vi "Icon Header.vi"(9 "Add Border? (F)":bool, 10 "BG (0=Random)":u32(colorbox), 11 "Text":string) -> (2 "BG out":u32(colorbox), 3 "Color256":T1)   [LabVIEW 2018, in "Pkg.lvlib"]
uses:
  Pkg.lvlib
  <vilib>/picture/picture.llb/imagedata.ctl
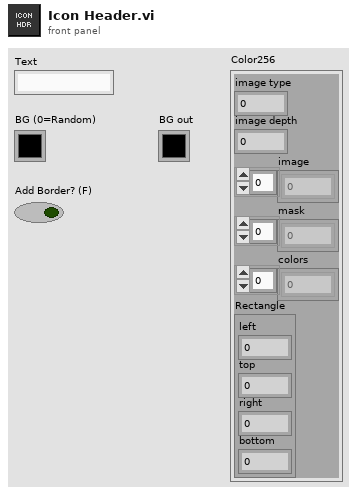
[diagram p1: front panel]
types:
  T1 = typedef "imagedata.ctl" = cluster{"image type":i32, "image depth":i32, "image":u8[], "mask":u8[], "colors":u32[], "Rectangle":cluster{"left":i16, "top":i16, "right":i16, "bottom":i16}}
  T2 = cluster{"left":i16, "top":i16, "right":i16, "bottom":i16}
  T3 = cluster{"Font Name:":string, "Size":i16, "Strikeout?":bool, "Italic?":bool, "Underline?":bool, "Outline?":bool, "Shadow?":bool, "Bold?":bool}
  T4 = enum16{"User-specified Font", "Application Font", "System Font", "Dialog Font"}
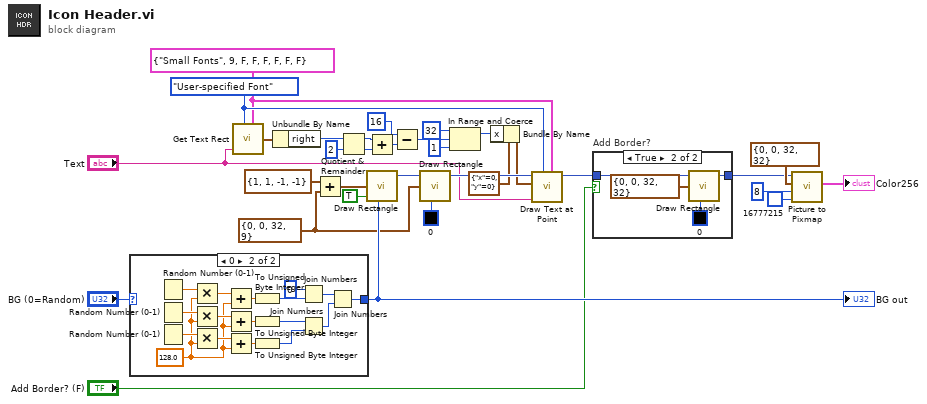
[diagram p0: block diagram]
diagram:
  w23 = T2 {"left"=0, "top"=0, "right"=32, "bottom"=9} ("rect")
  w20 = T3 {"Font Name:"="Small Fonts", "Size"=9, "Strikeout?"=FALSE, "Italic?"=FALSE, "Underline?"=FALSE, "Outline?"=FALSE, "Shadow?"=FALSE, "Bold?"=FALSE} ("[user-specified font]")
  w21 = T4."User-specified Font" ("desired font(Application)")
  n1 = case shown="0" "BG (0=Random)" {
    selector: "BG (0=Random)" -> [w33 _]
    tunnel: [w33 w38] -> w28
    frame Default {
    }
    frame 0 {
      w34 = 128.0 ("y")
      n2 = Random Number (0-1)() -> (number: 0 to 1=w49:dbl)
      n3 = Random Number (0-1)() -> (number: 0 to 1=w48:dbl)
      n4 = Random Number (0-1)() -> (number: 0 to 1=w45:dbl)
      n5 = Multiply(x=w49, y=w34) -> (x*y=w50:dbl)
      n6 = Multiply(x=w48, y=w34) -> (x*y=w47:dbl)
      n7 = Multiply(x=w45, y=w34) -> (x*y=w46:dbl)
      n8 = Add(x=w50, y=w34) -> (x+y=w35:dbl)
      n9 = Add(x=w47, y=w34) -> (x+y=w36:dbl)
      n10 = Add(x=w46, y=w34) -> (x+y=w37:dbl)
      n11 = To Unsigned Byte Integer(number=w35) -> (unsigned 8bit integer=w44:u8)
      n12 = To Unsigned Byte Integer(number=w36) -> (unsigned 8bit integer=w42:u8)
      n13 = To Unsigned Byte Integer(number=w37) -> (unsigned 8bit integer=w41:u8)
      n14 = Join Numbers(hi=u8 0, lo=w44) -> ((hi.lo)=w39:u16)
      n15 = Join Numbers(hi=w42, lo=w41) -> ((hi.lo)=w40:u16)
      n16 = Join Numbers(hi=w39, lo=w40) -> ((hi.lo)=w38:u32)
    }
  }
  "BG out" <- w28
  n17 = call <vilib>:"Get Text Rect.vi"("desired font(Application)"=w21, "text"="Text", "[user-specified font]"=w20) -> ("rect"=w19:T2)  [unwired: 6 in]
  n18 = Unbundle By Name(w19) -> ("right"=w9:i16)
  n19 = Add(x=T2 {"left"=1, "top"=1, "right"=-1, "bottom"=-1} ("rect"), y=w23) -> (x+y=w24:T2)
  n20 = Quotient & Remainder(x=w9, y=i16 2) -> (x-y*floor(x/y)=w6:i16, floor(x/y)=w12:i16)
  n21 = Add(x=w6, y=w12) -> (x+y=w7:i16)
  n22 = call <vilib>:"Draw Rectangle.vi"("rect"=w24, "fill?(F)"=TRUE, "color(black)"=w28) -> ("new picture"=w30:picture)  [unwired: 6 in]
  n23 = Subtract(x=i16 16 ("y"), y=w7) -> (x-y=w5:i16)
  n24 = call <vilib>:"Draw Rectangle.vi"("picture"=w30, "rect"=w23, "color(black)"=u32 0) -> ("new picture"=w22:picture)  [unwired: 6 in]
  n25 = In Range and Coerce(upper limit=i16 32, x=w5, lower limit=i16 1) -> (coerced(x)=w11:i16)  [unwired: 1 out]
  n26 = Bundle By Name(cluster=cluster{"x":i16, "y":i16} {"x"=0, "y"=0} ("origin"), "x"=w11) -> (w16:cluster{"x":i16, "y":i16})
  n27 = call <vilib>:"Draw Text at Point.vi"("[user-specified font]"=w20, "desired font(Application)"=w21, "text"="Text", "origin"=w16, "picture"=w22) -> ("new picture"=w4:picture)  [unwired: 5 in, 1 out]
  n28 = case "Add Border?" shown="True" "Add Border? (F)" {
    tunnel: w4 -> [w51 w54]
    tunnel: [w51 w53] -> w3
    frame False {
    }
    frame True {
      n29 = call <vilib>:"Draw Rectangle.vi"("picture"=w54, "rect"=T2 {"left"=0, "top"=0, "right"=32, "bottom"=32}, "color(black)"=u32 0) -> ("new picture"=w53:picture)  [unwired: 6 in]
    }
  }
  n30 = call <vilib>:"Picture to Pixmap.vi"("Background Color"=u32 16777215, "depth"=8, "rect"=T2 {"left"=0, "top"=0, "right"=32, "bottom"=32}, "picture"=w3) -> ("image data"=→"Color256":T1)  [unwired: 6 in, 1 out]
